vi "axex_get_workbook.vi"(8 "error in":errorcluster, 9 "open active workbook (False)":bool, 10 "reload from file (False)":bool, 11 "AX Excel instance in":T1) -> (0 "error out":errorcluster, 2 "excel workbook":refnum<k7>, 3 "AX Excel instance out":T1)   [LabVIEW 2020, in "AX Excel.lvlib"]
doc: "Get reference to excel workbook (file) by file name. If the file of the given name is not loaded in Excel it will be opened from the disk.\nIf 'reload from file' is true and the file is already opened in Excel it will be closed WITHOUT SAVING changes and it will be reloaded from disk again.\nDon't close returned reference, it remains opened in SX Excel instance handle until file is closed!"
uses:
  AX Excel.lvlib
  axex_instance.ctl
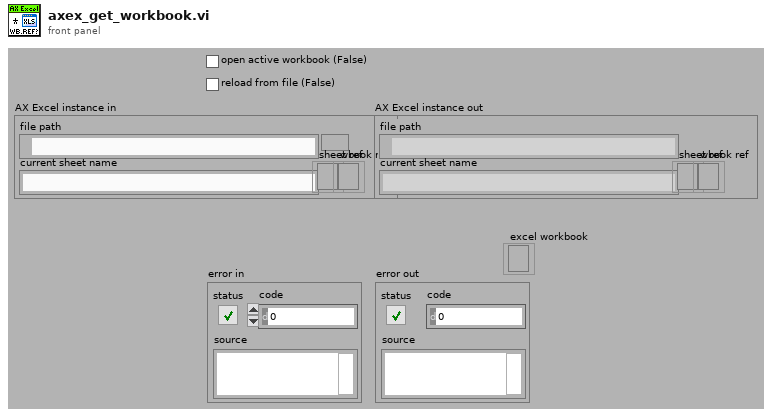
[diagram p1: front panel]
types:
  T1 = typedef "AX Excel.lvlib/axex_instance.ctl" = cluster{"file path":path, "current sheet name":string, "sheet ref":refnum<k7>, "wbook ref":refnum<k7>}
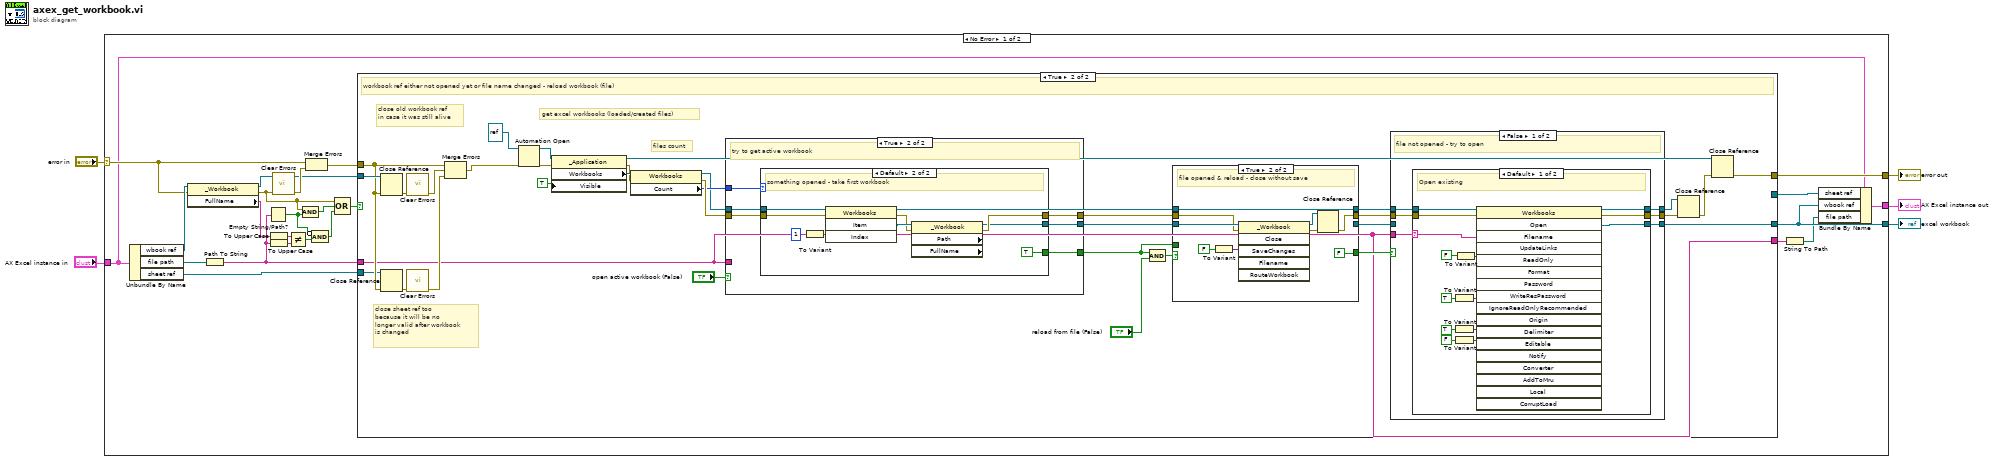
[diagram p0: block diagram]
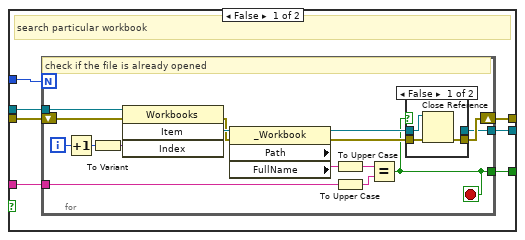
[diagram p3: hidden frame]
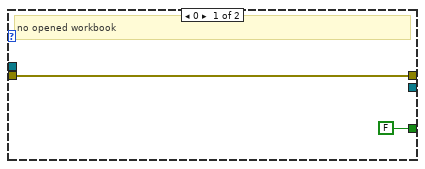
[diagram p5: hidden frame]
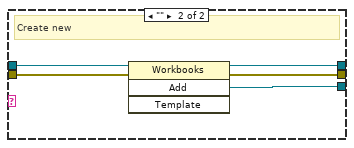
[diagram p7: hidden frame]
diagram:
  n1 = case shown="No Error" "error in" {
    selector: "error in" -> [w19 w155]
    tunnel: [w29 w155] -> w5
    tunnel: [w10 _] -> w3
    tunnel: "AX Excel instance in" -> [w12 w154]
    tunnel: [w11 w154] -> w1
    frame No Error {
      n2 = Unbundle By Name(w12) -> ("wbook ref"=w28:refnum<k7>, "file path"=w26:path, "sheet ref"=w8:refnum<k7>)
      n3 = property class="_Workbook"(reference=w28, error in=w19) -> (reference out=w16:refnum<k7>, error out=w18:errorcluster, "FullName"=w25:string)
      n4 = Path To String(path=w26) -> (string=w20:string)
      n5 = Empty String/Path?(string/path=w20) -> (empty?=w14:bool)
      n6 = To Upper Case(1:w25) -> (0:w21:string)
      n7 = To Upper Case(1:w20) -> (0:w24:string)
      n8 = call <vilib>:"Clear Errors.vi"("error in (no error)"=w18) -> ("error out"=w22:errorcluster)  [unwired: 5 in, 1 out]
      n9 = Not Equal?(x=w21, y=w24) -> (x != y?=w15:bool)
      n10 = Compound Arithmetic op=AND(w18, w14) -> (w17:bool)
      n11 = Merge Errors(w19, w22) -> (w27:errorcluster)
      n12 = Compound Arithmetic op=AND(invert w14, w15) -> (w13:bool)
      n13 = Compound Arithmetic op=OR(w18, w17, w13) -> (w23:bool)
      n14 = case shown="True" w23 {
        tunnel: w27 -> [w31 w41]
        tunnel: [w31 w58] -> w29
        tunnel: [w32 w57] -> w10
        tunnel: w20 -> [w30 w34]
        tunnel: w16 -> [w32 w43]
        tunnel: [w33 _] -> w9
        tunnel: w8 -> [w33 w38]
        tunnel: [w30 w34] -> w7
        frame False {
          # "workbook reference is alive && (file name match || no filename given) - return current workbook reference"
        }
        frame True {
          # "close sheet ref too\nbecause it will be no\nlonger valid after workbook\nis changed"
          # "close old workbook ref\nin case it was still alive"
          # "files count"
          # "get excel workbooks (loaded/created files)"
          # "workbook ref either not opened yet or file name changed - reload workbook (file)"
          n15 = Close Reference(reference=w43, error in (no error)=w41) -> (error out=w45:errorcluster)
          n16 = Close Reference(reference=w38, error in (no error)=w41) -> (error out=w40:errorcluster)
          n17 = call <vilib>:"Clear Errors.vi"("error in (no error)"=w45) -> ("error out"=w44:errorcluster)  [unwired: 5 in, 1 out]
          n18 = call <vilib>:"Clear Errors.vi"("error in (no error)"=w40) -> ("error out"=w39:errorcluster)  [unwired: 5 in, 1 out]
          n19 = Merge Errors(w41, w44, w39) -> (w42:errorcluster)
          n20 = Automation Open(error in (no error)=w42, Automation Refnum=refnum<k7> refnum ("Excel._Application")) -> (Automation Refnum=w37:refnum<k7>, error out=w67:errorcluster)  [unwired: 2 in]
          n21 = property class="_Application"(reference=w37, error in=w67, "Visible"=TRUE) -> (reference out=w66:refnum<k7>, error out=w60:errorcluster, "Workbooks"=w63:refnum<k7>)
          n22 = property class="Workbooks"(reference=w63, error in=w60) -> (reference out=w52:refnum<k7>, error out=w65:errorcluster, "Count"=w64:i32)
          n23 = case shown="True" "open active workbook (False)" {
            tunnel: w65 -> [w74 w100]
            tunnel: w64 -> [w73 w98]
            tunnel: [w72 w96] -> w56
            tunnel: [w71 w99] -> w54
            tunnel: w52 -> [w70 w101]
            tunnel: [w69 w97] -> w47
            tunnel: w34 -> [w68 _]
            frame False {
              # "search particular workbook"
              n24 = for {
                N: w73 -> [_]
                shift-right: [w79] -> w71
                shift-left: w74 -> [w89]
                tunnel: w70 -> [w87]
                tunnel: w68 -> [w80]
                tunnel: [w78] -> w72
                tunnel: [w77] -> w69
                i -> [w85]
                stop <- w77 stop-if-true
                # "check if the file is already opened"
                n25 = Increment(x=w85) -> (x+1=w84:i32)
                n26 = To Variant(anything=w84) -> (Variant=w86:variant)
                n27 = invoke class="Workbooks" method="Item"(reference=w87, error in=w89, "Index"=w86) -> (error out=w88:errorcluster, "Item"=w90:refnum<k7>)  [unwired: 1 in, 2 out]
                n28 = property class="_Workbook" props=["Path", "FullName"](reference=w90, error in=w88) -> (reference out=w82:refnum<k7>, error out=w83:errorcluster, "FullName"=w81:string)  [unwired: 1 out]
                n29 = To Upper Case(1:w81) -> (0:w76:string)
                n30 = To Upper Case(1:w80) -> (0:w75:string)
                n31 = Equal?(x=w76, y=w75) -> (x = y?=w77:bool)
                n32 = case shown="False" w77 {
                  tunnel: w83 -> [w93 w95]
                  tunnel: w82 -> [w91 w94]
                  tunnel: [w92 w95] -> w79
                  tunnel: [_ w94] -> w78
                  frame False {
                    n33 = Close Reference(reference=w91, error in (no error)=w93) -> (error out=w92:errorcluster)
                  }
                  frame True {
                  }
                }
              }
            }
            frame True {
              # "try to get active workbook"
              n34 = case shown="Default" w98 {
                tunnel: w101 -> [_ w111]
                tunnel: w100 -> [w103 w110]
                tunnel: [w103 w106] -> w99
                tunnel: [FALSE ("Visible") TRUE ("Visible")] -> w97
                tunnel: [_ w104] -> w96
                frame 0 {
                  # "no opened workbook"
                }
                frame Default {
                  # "something opened - take first workbook"
                  n35 = To Variant(anything=1) -> (Variant=w112:variant)
                  n36 = invoke class="Workbooks" method="Item"(reference=w111, error in=w110, "Index"=w112) -> (error out=w107:errorcluster, "Item"=w108:refnum<k7>)  [unwired: 1 in, 2 out]
                  n37 = property class="_Workbook" props=["Path", "FullName"](reference=w108, error in=w107) -> (reference out=w104:refnum<k7>, error out=w106:errorcluster)  [unwired: 2 out]
                }
              }
            }
          }
          n38 = Compound Arithmetic op=AND(w47, "reload from file (False)") -> (w49:bool)
          n39 = case shown="True" w49 {
            tunnel: [w115 _] -> w55
            tunnel: w56 -> [w115 w124]
            tunnel: [w114 w120] -> w53
            tunnel: w54 -> [w114 w123]
            tunnel: w52 -> [w116 w125]
            tunnel: [w116 w125] -> w51
            tunnel: [w113 FALSE] -> w50
            tunnel: w47 -> [w113 _]
            frame False {
            }
            frame True {
              # "file opened & reload - close without save"
              n40 = To Variant(anything=FALSE) -> (Variant=w117:variant)
              n41 = invoke class="_Workbook" method="Close"(reference=w124, error in=w123, "SaveChanges"=w117) -> (reference out=w121:refnum<k7>, error out=w122:errorcluster)  [unwired: 3 in, 4 out]
              n42 = Close Reference(reference=w121, error in (no error)=w122) -> (error out=w120:errorcluster)
            }
          }
          n43 = case shown="False" w50 {
            tunnel: w51 -> [w131 w152]
            tunnel: w53 -> [w130 w153]
            tunnel: w34 -> [w126 _]
            tunnel: [w129 w153] -> w62
            tunnel: [w128 w152] -> w61
            tunnel: [w127 w151] -> w57
            tunnel: w55 -> [_ w151]
            frame False {
              # "file not opened - try to open"
              n44 = case shown="Default" w126 {
                selector: w126 -> [w132 _]
                tunnel: w131 -> [w145 w150]
                tunnel: w130 -> [w144 w149]
                tunnel: [w137 w148] -> w129
                tunnel: [w136 w147] -> w128
                tunnel: [w135 w146] -> w127
                frame Default {
                  # "Open existing"
                  n45 = To Variant(anything=TRUE) -> (Variant=w133:variant)
                  n46 = To Variant(anything=TRUE) -> (Variant=w140:variant)
                  n47 = To Variant(anything=FALSE) -> (Variant=w141:variant)
                  n48 = To Variant(anything=FALSE) -> (Variant=w139:variant)
                  n49 = invoke class="Workbooks" method="Open"(reference=w145, error in=w144, "Filename"=w132, "ReadOnly"=w139, "IgnoreReadOnlyRecommended"=w133, "Editable"=w140, "Notify"=w141) -> (reference out=w136:refnum<k7>, error out=w137:errorcluster, "Open"=w135:refnum<k7>)  [unwired: 11 in, 15 out]
                }
                frame "" {
                  # "Create new"
                  n50 = invoke class="Workbooks" method="Add"(reference=w150, error in=w149) -> (reference out=w147:refnum<k7>, error out=w148:errorcluster, "Add"=w146:refnum<k7>)  [unwired: 2 in, 1 out]
                }
              }
            }
            frame True {
              # "file already opened - do nothing"
            }
          }
          n51 = Close Reference(reference=w61, error in (no error)=w62) -> (error out=w59:errorcluster)
          n52 = Close Reference(reference=w66, error in (no error)=w59) -> (error out=w58:errorcluster)
        }
      }
      n53 = String To Path(string=w7) -> (path=w6:path)
      n54 = Bundle By Name(cluster=w12, "sheet ref"=w9, "wbook ref"=w10, "file path"=w6) -> (w11:T1)
    }
    frame Error {
    }
  }
  "error out" <- w5
  "excel workbook" <- w3
  "AX Excel instance out" <- w1
